vi "ComputeMean.vi"(10 "Array In":dbl[](array[numeric]), 11 "No. of Readings":i32) -> (3 "Mean":dbl)   [LabVIEW 2019]
panel:
  out "Numeric":i32
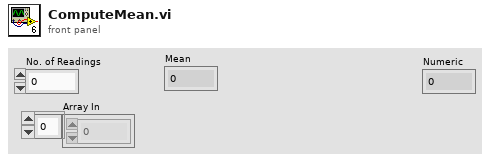
[diagram p1: front panel]
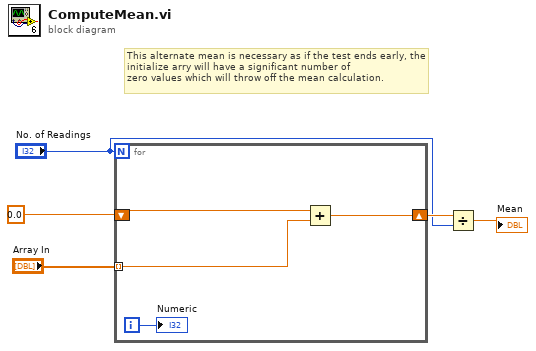
[diagram p0: block diagram]
diagram:
  # "This alternate mean is necessary as if the test ends early, the initialize arry will have a significant number of \nzero values which will throw off the mean calculation."
  n1 = for {
    N: "No. of Readings" -> [_]
    tunnel: "Array In" -> [w9] mode=indexing
    shift-right: [w7] -> w3
    shift-left: 0.0 -> [w8]
    i -> [w6]
    n2 = Add(x=w8, y=w9) -> (x+y=w7:dbl)
    "Numeric" <- w6
  }
  n3 = Divide(x=w3, y="No. of Readings") -> (x/y=→"Mean":dbl)
